vi "get velocity-scaled.vi"(9 "Array":string[](array[string]), 10 "Array 2":refnum<vi>[](array[refnum]), 11 "MulticolumnListbox in":refnum<vi>) -> (0 "error out":errorcluster, 2 "Array 3":ext[](array[numeric]), 3 "Array 4":refnum<vi>[](array[refnum]))   [LabVIEW 2016, in "scale sub-VIs.lvlib"]
uses:
  sub-VIs/scale sub-VIs.lvlib
  <vilib>/Utility/miscctls.llb/LVRowAndColumnTypeDef.ctl
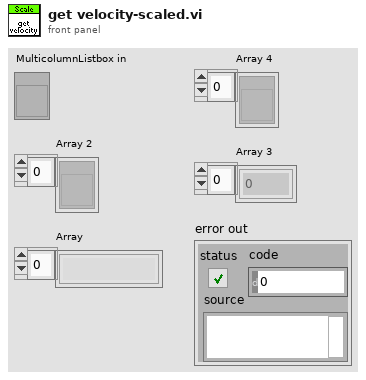
[diagram p1: front panel]
types:
  T1 = typedef "LVRowAndColumnTypeDef.ctl" = cluster{"Row":i32, "Column":i32}
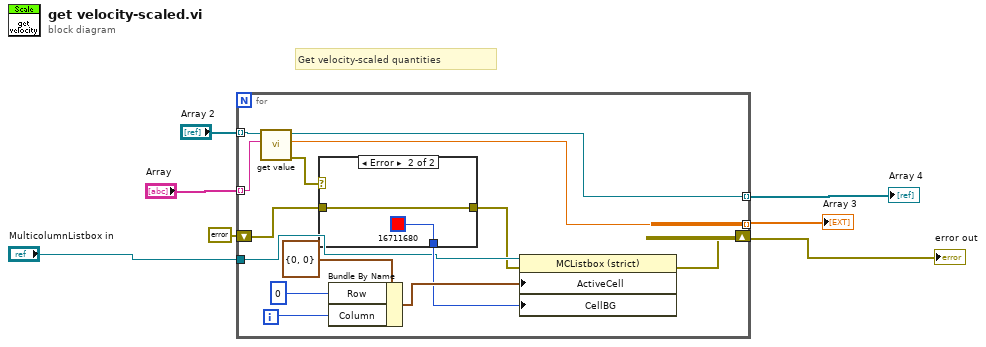
[diagram p0: block diagram]
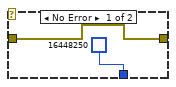
[diagram p2: hidden frame]
diagram:
  # "Get velocity-scaled quantities"
  n1 = for {
    tunnel: "Array" -> [w11] mode=indexing
    tunnel: "Array 2" -> [w21] mode=indexing
    tunnel: [w20] -> w2 mode=indexing
    tunnel: [w19] -> w3 mode=indexing
    shift-right: [w8] -> w6
    shift-left: errorcluster {"status"=FALSE, "code"=0, "source"=""} ("error IO") -> [w13]
    tunnel: "MulticolumnListbox in" -> [w10]
    i -> [w16]
    n2 = call "get value.vi"("Control Name"=w11, "VI Refnum"=w21) -> ("error out"=w14:errorcluster, "get value"=w19:ext, "VI Refnum out"=w20:refnum<vi>)  [unwired: 7 in]
    n3 = case shown="Error" w14 {
      tunnel: [u32 16448250 u32 16711680] -> w15
      tunnel: [w22 w24] -> w9
      tunnel: w13 -> [w22 w24]
      frame No Error {
      }
      frame Error {
      }
    }
    n4 = Bundle By Name(cluster=T1 {"Row"=0, "Column"=0} ("Active Cell:Active Cell"), "Row"=0, "Column"=w16) -> (w17:T1)
    n5 = property on="Property Node" class="MCListbox (strict)"(reference=w10, error in=w9, "ActiveCell"=w17, "CellBG"=w15) -> (error out=w8:errorcluster)  [unwired: 1 out]
  }
  "error out" <- w6
  "Array 3" <- w3
  "Array 4" <- w2
